vi "Target.vi"() -> ()   [LabVIEW 2018]
uses:
  <vilib>/Platform/TimedLoop/XDataNode/timing_clust.ctl
  <vilib>/Platform/TimedLoop/XDataNode/nitl_modes.ctl
  <vilib>/Platform/TimedLoop/XDataNode/wakeup.ctl
  <vilib>/rvi/eio/common/nirviEmuTemplateMethod_errors.vi
  <vilib>/rvi/Emulation/niFpgaGetClockAttributes.vi
  <vilib>/rvi/Emulation/niFpgaSctlEmulationGetInTimedLoop.vi
  <vilib>/rvi/Emulation/niFpgaEmulationReportErrorSimple.vi
  <vilib>/rvi/Emulation/niFpgaCriticalErrorInLSC.vi
  <vilib>/rvi/Emulation/niFpgaProcessEmulError.vi
  <vilib>/rvi/DataTransferAndStorage/Container/Common/niFpgaContainerGetUniqueNameForEmu.vi
  <vilib>/rvi/interface/RandomDataEmulation/niFpgaRandomDataHandleErrors.vi
  <vilib>/rvi/Memory/Memory_Emulation/niFpgaMemoryFastEmulationDramWriteAndRequestData.vi
  <vilib>/rvi/Memory/Memory_Emulation/niFpgaMemoryEmulationDramWriteAndRequestData.vi
  <vilib>/rvi/Memory/Memory_Emulation/niFpgaMemoryEmulationDramWriteAndRequestDataApplyByteEnables.vi
  <vilib>/eio/EIONode/EIONode.xnode
  <vilib>/Platform/TimedLoop/XDataNode/XDataNode.xnode
  <vilib>/rvi/DataTransferAndStorage/Container/XNode/niFpgaContainer.xnode
  <vilib>/rvi/Memory/Memory_Emulation/niFpgaMemoryEmulationDramRetrieveData.vi
  <vilib>/rvi/interface/RandomDataEmulation/nirviRandomDataFpgaReadWriteTemplate.vi
  <vilib>/Platform/TimedLoop/XDataNode/XDNodeRunTimeDep.lvlib
panel:
  in  "TrigTime":u32=500
  in  "ForcedStopMemory":bool
  out "CountFIFO":u32
  out "AddCounter":u32
  in  "9..0(F)/0..9(T)":bool
  in  "Retrieve":u8=1
  in  "Request":u8
  in  "ResetFIFO":bool
  out "FIFOIsDone":bool
  in  "ResetMemory":bool
  out "MemoryIsDone":bool
  in  "LastAdd":u32=81920
  in  "FirstAdd":u32
  in  "MemoryToFIFO":bool
  in  "DataToMemory":bool
  in  "NumberOfAdd":u32=1310720
  in  "18_STOP":u8=18
  in  "26_STOP":u8=26
  in  "TRIG":bool
  in  "Такт чтения после адреса":u8
  in  "Чтение по С(F)/Ф(T)":bool
  in  "CSN в конце по С(F)/Ф(T)":bool
  in  "ResetSPI":bool
  out "SPI_is_done":bool
  in  "Делитель 24/x":u8=2
  in  "Автомат":bool
  in  "RESET":bool
  out "MISO":bool[](array[boolean])
  in  "MOSI":bool[](array[boolean])=[FALSE, FALSE, FALSE, FALSE, FALSE, FALSE, FALSE, FALSE, FALSE, FALSE, FALSE, FALSE, FALSE, FALSE, FALSE, FALSE, FALSE, FALSE, FALSE, FALSE, FALSE, FALSE, FALSE, FALSE]
  in  "SPI":bool
  in  "8-bit(F)/16-bit(T)":bool
  in  "Stop_FPGA":bool
  # "0"
  # "0"
  # "7"
  # "7"
  # "Начало слова (8 bit)"
  # "Конец адреса (8 bit)"
  # "8"
  # "Начало адреса (8 bit)"
  # "14"
  # "15"
  # "R(F)/W(T) (8 bit)"
  # "Начало слова (16 bit)"
  # "15"
  # "Конец адреса (16 bit)"
  # "16"
  # "Начало адреса (16 bit)"
  # "22"
  # "R(F)/W(T) (16 bit)"
  # "23"
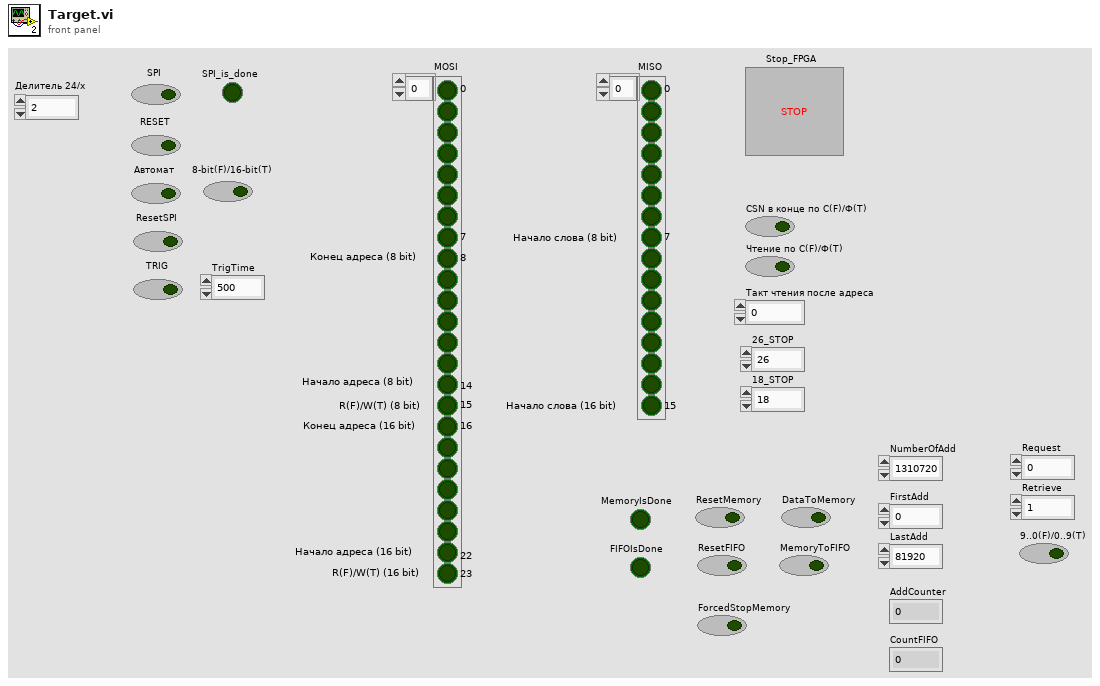
[diagram p1: front panel]
types:
  T1 = typedef "XDNodeRunTimeDep.lvlib/timing_clust.ctl" = cluster{"Expected End [f-1]":u64, "Actual End [f-1]":u64, "Finished Late? [f-1]":bool, "Expected End [i-1]":u64, "Actual End [i-1]":u64, "Finished Late? [i-1]":bool, "Expected Start [i]":u64, "Actual Start [i]":u64, "Expected Start [f]":u64, "Actual Start [f]":u64, "Source Name":string, "Structure Name":string, "Period":i64, "Deadline":i64, "Offset":i64, "Start":i64, "Priority":i32, "Timeout":i32, "Mode":T2, "Wakeup Reason":T3, "Error":errorcluster, "Source Type":string, "Secondary Source Type":string, "Global End Time":u64, "Global Start Time":u64, "Frame Duration":u64, "Iteration Duration":u64, "Assigned CPU":i32, "I/O Scan Engine Mode":u32}
  T2 = typedef "XDNodeRunTimeDep.lvlib/nitl_modes.ctl" = enum32{"No Change", "Process missed periods, maintain original phase", "Discard missed periods, maintain original phase", "Process missed periods, ignore original phase", "Discard missed periods, ignore original phase"}
  T3 = typedef "XDNodeRunTimeDep.lvlib/wakeup.ctl" = enum32{"Normal", "Aborted", "Asynchronous wakeup", "Timing source error", "Timed loop error", "Timeout"}
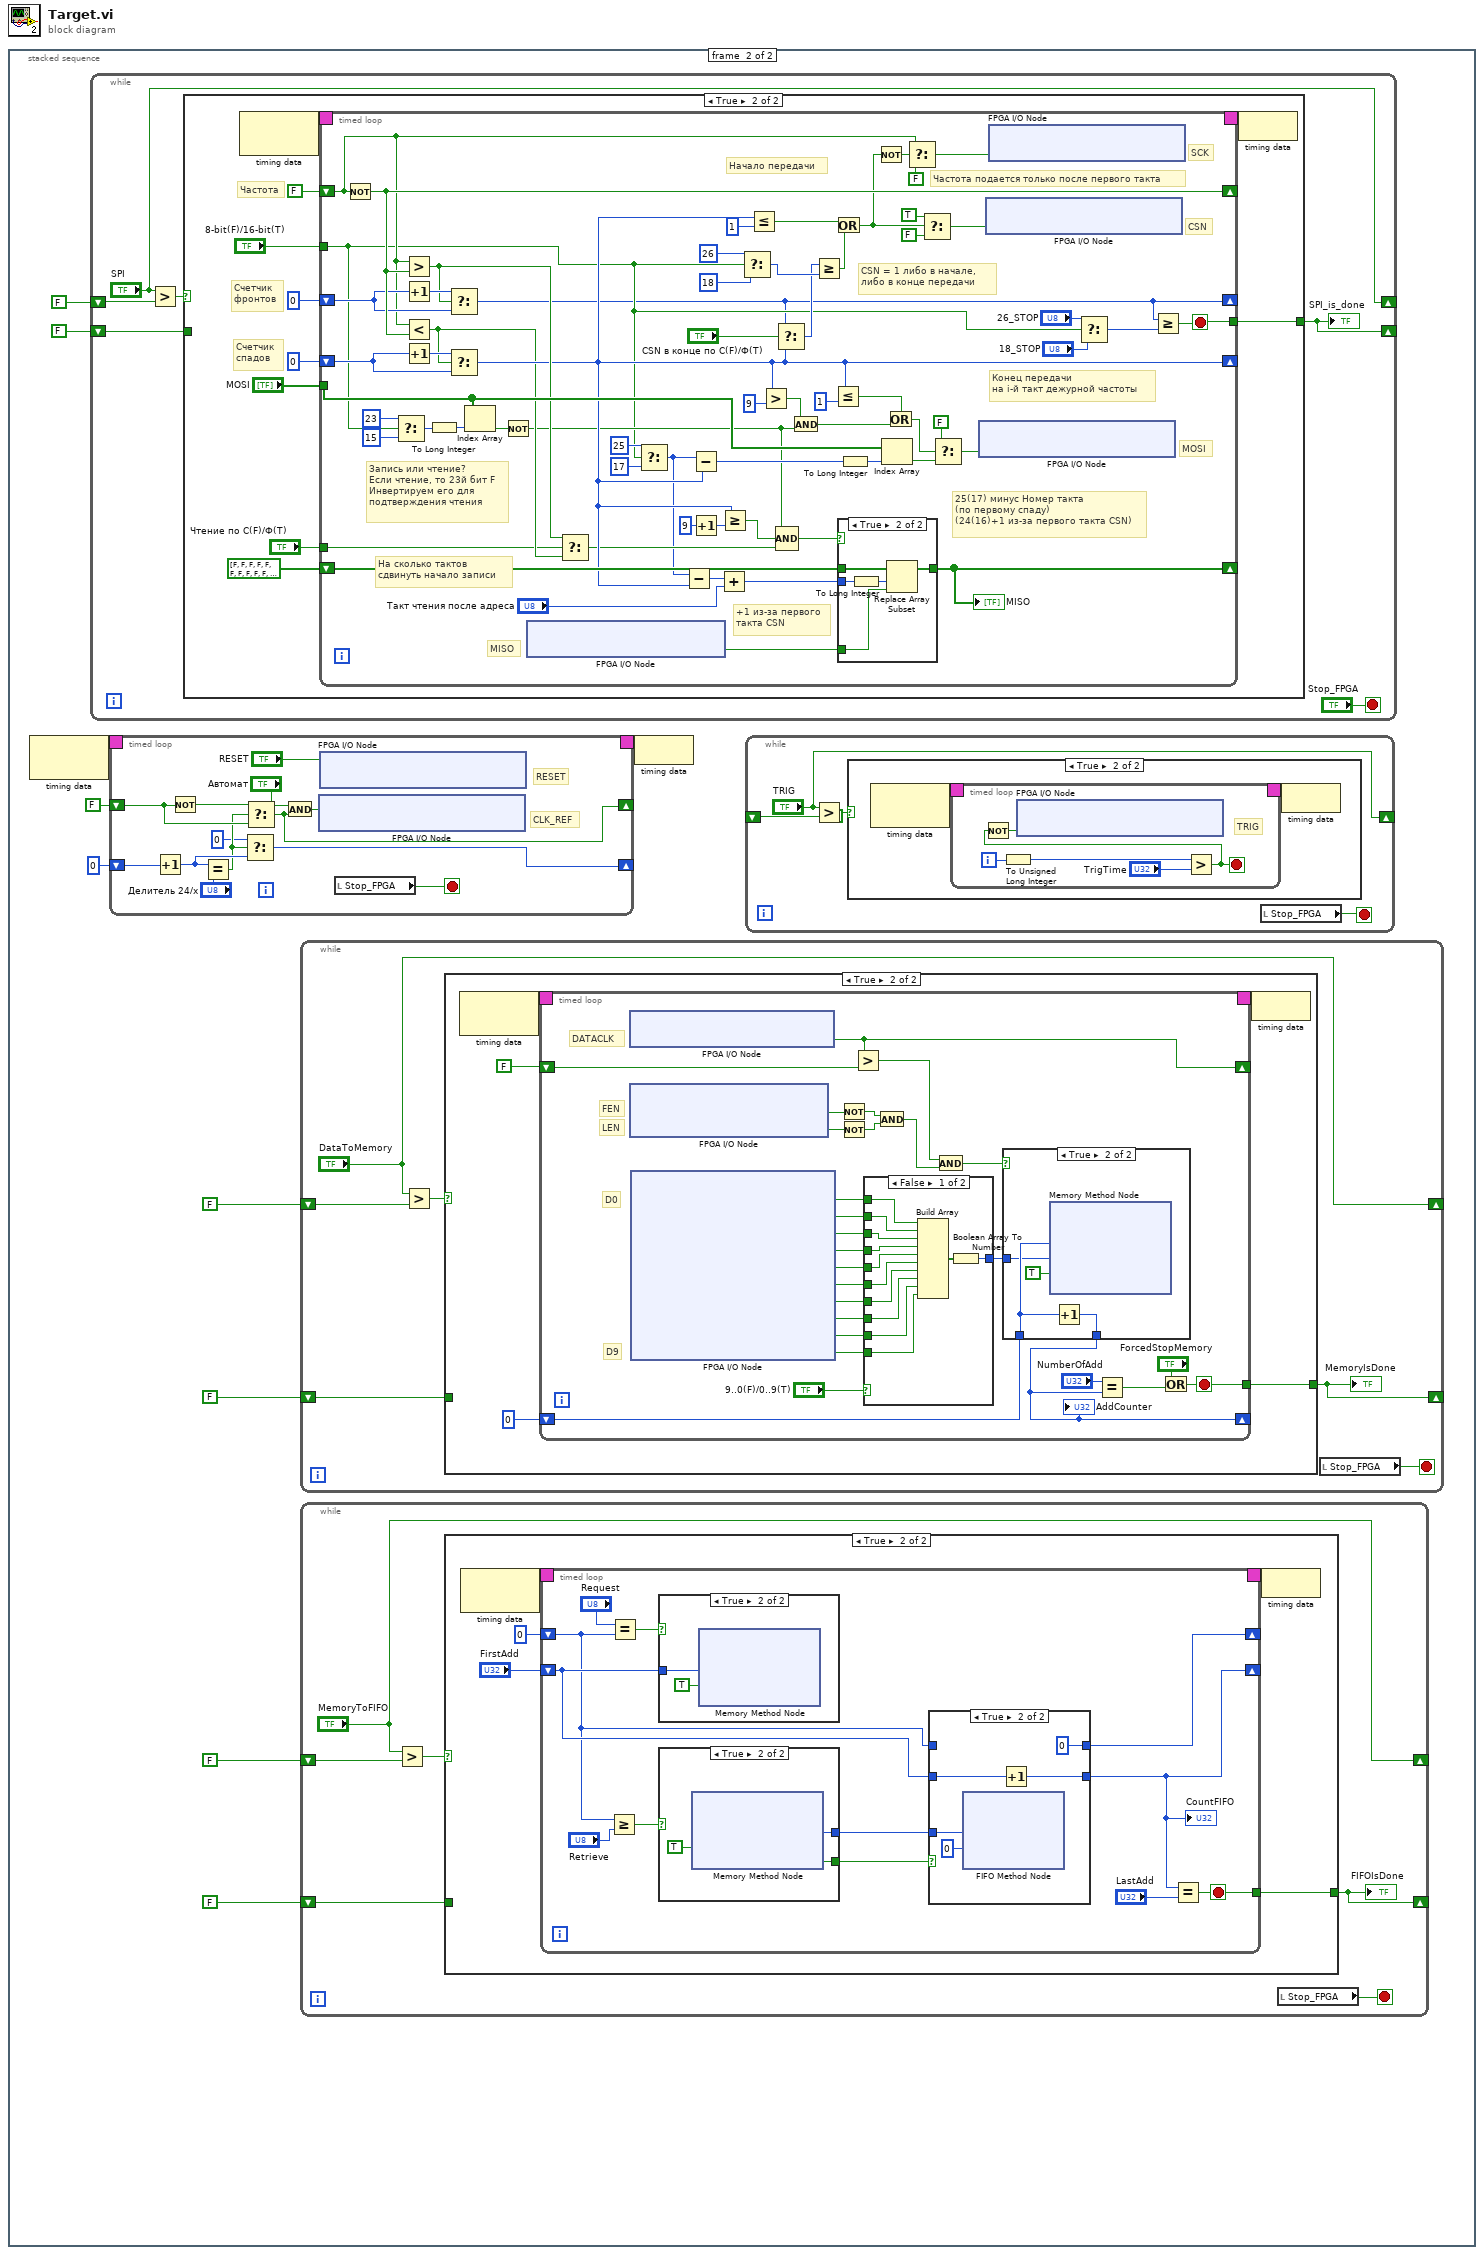
[diagram p0: block diagram]
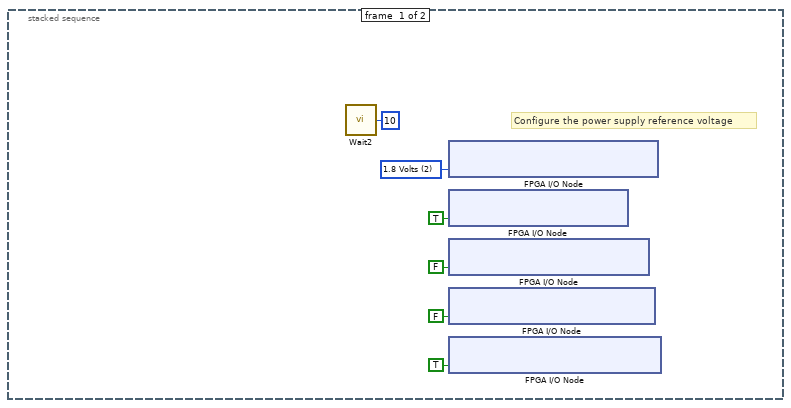
[diagram p2: hidden frame]
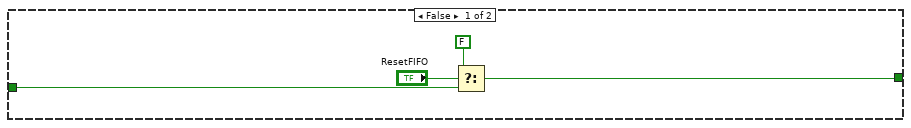
[diagram p4: hidden frame]
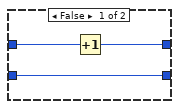
[diagram p5: hidden frame]
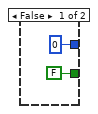
[diagram p6: hidden frame]
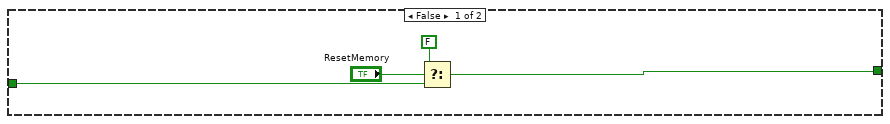
[diagram p8: hidden frame]
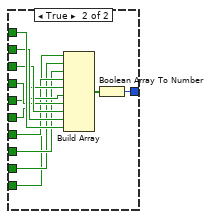
[diagram p9: hidden frame]
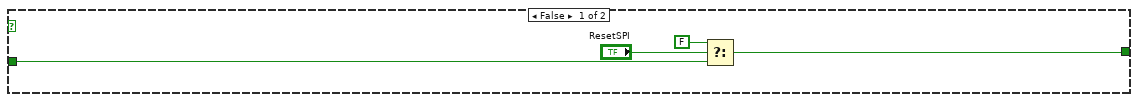
[diagram p11: hidden frame]
diagram:
  n1 = stacked-sequence {
    frame #0 {
      w6 = u8 2 items=["3.3 Volts", "2.5 Volts", "1.8 Volts"] ("Internal Power Supply Voltage")
      # "Configure the power supply reference voltage"
      n2 = call "Wait2"("Count(mSec)"=u8 10) -> ()  [unwired: 1 out]
      n3 = xnode "FPGA I/O Node"("IO Module\\Local_Supply_Select"=w6) -> ()  [unwired: 1 in, 1 out]
      n4 = xnode "FPGA I/O Node"("IO Module\\DDCA_PFI_WE"=TRUE ("IO Module\\DDCB_PFI_WE")) -> ()  [unwired: 1 in, 1 out]
      n5 = xnode "FPGA I/O Node"("IO Module\\DDCA_DIO0-7_WE"=FALSE ("IO Module\\DDCA_DIO0-7_WE")) -> ()  [unwired: 1 in, 1 out]
      n6 = xnode "FPGA I/O Node"("IO Module\\DDCA_DIO8-15_WE"=FALSE ("IO Module\\DDCA_DIO8-15_WE")) -> ()  [unwired: 1 in, 1 out]
      n7 = xnode "FPGA I/O Node"("IO Module\\DDCA_DIO16-23_WE"=TRUE ("IO Module\\DDCA_DIO16-23_WE")) -> ()  [unwired: 1 in, 1 out]
    }
    frame #1 {
      n8 = node-c288() -> (w16:T1)  [unwired: 1 in]
      n9 = while {
        shift-right: ["SPI"] -> _
        shift-left: FALSE -> [w176]
        shift-right: [w171] -> _
        shift-left: FALSE -> [w172]
        stop <- "Stop_FPGA" stop-if-true
        n10 = Greater?(x="SPI", y=w176) -> (0:w175:bool)
        n11 = case shown="True" w175 {
          tunnel: [w179 w185] -> w171
          tunnel: w172 -> [w177 _]
          frame False {
            n12 = Select(t=FALSE, s="ResetSPI", f=w177) -> (s? t:f=w179:bool)
          }
          frame True {
            # "Счетчик\nфронтов"
            # "Счетчик\nспадов"
            # "Частота"
            n13 = node-c288() -> (w190:T1)  [unwired: 1 in]
            n14 = timed-loop {
              timing: w190 -> [_]
              timing-out: [_] -> w189
              shift-right: [w196] -> _
              shift-left: u8 0 -> [w249]
              shift-right: [w252] -> _
              shift-left: FALSE -> [w244]
              shift-right: [w219] -> _
              shift-left: u8 0 -> [w250]
              tunnel: [w195] -> w185
              tunnel: "8-bit(F)/16-bit(T)" -> [w198]
              shift-right: [w233] -> _
              shift-left: bool[] [FALSE, FALSE, FALSE, FALSE, FALSE, FALSE, FALSE, FALSE, FALSE, FALSE, FALSE, FALSE, FALSE, FALSE, FALSE, FALSE] -> [w234]
              tunnel: "MOSI" -> [w228]
              tunnel: "Чтение по С(F)/Ф(T)" -> [w204]
              stop <- w195 stop-if-true
              # "MISO"
              # "MOSI"
              # "CSN"
              # "SCK"
              # "На сколько тактов \ncдвинуть начало записи"
              # "25(17) минус Номер такта\n(по первому спаду)\n(24(16)+1 из-за первого такта CSN)"
              # "Запись или чтение?\nЕсли чтение, то 23й бит F\nИнвертируем его для\nподтверждения чтения"
              # "+1 из-за первого\nтакта CSN"
              # "Конец передачи\nна i-й такт дежурной частоты"
              # "Начало передачи"
              # "Частота подается только после первого такта"
              # "CSN = 1 либо в начале,\nлибо в конце передачи"
              n15 = Not(x=w244) -> (.not. x?=w252:bool)
              n16 = Select(t=u8 23, s=w198, f=u8 15) -> (s? t:f=w241:u8)
              n17 = Greater?(x=w244, y=w252) -> (0:w222:bool)
              n18 = Increment(x=w249) -> (x+1=w253:u8)
              n19 = Less?(x=w244, y=w252) -> (x < y?=w214:bool)
              n20 = Increment(x=w250) -> (x+1=w251:u8)
              n21 = To Long Integer(number=w241) -> (32bit integer=w240:i32)
              n22 = Select(t=w253, s=w222, f=w249) -> (s? t:f=w196:u8)
              n23 = Select(t=w251, s=w214, f=w250) -> (s? t:f=w219:u8)
              n24 = Index Array(array=w228, index=w240) -> (element=w218:bool)
              n25 = Not(x=w218) -> (.not. x?=w212:bool)
              n26 = xnode "FPGA I/O Node"() -> ("IO Module\\DDCA_DIO0_Read"=w191:bool)  [unwired: 1 in, 1 out]
              n27 = Select(t=w222, s=w204, f=w214) -> (s? t:f=w213:bool)
              n28 = Select(t=u8 25 ("y"), s=w198, f=u8 17) -> (s? t:f=w209:u8)
              n29 = Subtract(x=w209, y=w219) -> (x-y=w203:u8)
              n30 = Subtract(x=w209, y=w219) -> (x-y=w221:u8)
              n31 = Increment(x=u8 9 ("Такт чтения")) -> (x+1=w215:u8)
              n32 = Add(x=w203, y="Такт чтения после адреса") -> (x+y=w220:u8)
              n33 = Greater Or Equal?(x=w219, y=w215) -> (x >= y?=w217:bool)
              n34 = Select(t=u8 26 ("Такт CSN в коцне"), s=w198, f=u8 18 ("Такт CSN в конце")) -> (s? t:f=w208:u8)
              n35 = Less Or Equal?(x=w219, y=u8 1 ("1")) -> (x <= y?=w245:bool)
              n36 = Greater?(x=w219, y=u8 9 ("18")) -> (0:w236:bool)
              n37 = Select(t=w196, s="CSN в конце по С(F)/Ф(T)", f=w219) -> (s? t:f=w207:u8)
              n38 = Compound Arithmetic op=AND(w212, w217, w213) -> (w237:bool)
              n39 = And(x=w236, y=w212) -> (x .and. y?=w232:bool)
              n40 = Greater Or Equal?(x=w207, y=w208) -> (x >= y?=w201:bool)
              n41 = Less Or Equal?(x=w219, y=u8 1 ("18")) -> (x <= y?=w230:bool)
              n42 = Or(x=w245, y=w201) -> (x .or. y?=w205:bool)
              n43 = case shown="True" w237 {
                tunnel: w220 -> [_ w259]
                tunnel: w234 -> [w254 w258]
                tunnel: [w254 w257] -> w233
                tunnel: w191 -> [_ w255]
                frame False {
                }
                frame True {
                  n44 = To Long Integer(number=w259) -> (32bit integer=w256:i32)
                  n45 = Replace Array Subset(array=w258, new element=w255, index=w256) -> (w257:bool[])
                }
              }
              "MISO" <- w233
              n46 = To Long Integer(number=w221) -> (32bit integer=w248:i32)
              n47 = Not(x=w205) -> (.not. x?=w206:bool)
              n48 = Index Array(array=w228, index=w248) -> (element=w239:bool)
              n49 = Or(x=w230, y=w232) -> (x .or. y?=w231:bool)
              n50 = Select(t=w244, s=w206, f=FALSE) -> (s? t:f=w194:bool)
              n51 = Select(t=TRUE, s=w205, f=FALSE) -> (s? t:f=w193:bool)
              n52 = Select(t=FALSE, s=w231, f=w239) -> (s? t:f=w192:bool)
              n53 = xnode "FPGA I/O Node"("IO Module\\DDCA_PFI3_Write"=w192) -> ()  [unwired: 1 in, 1 out]
              n54 = xnode "FPGA I/O Node"("IO Module\\DDCA_PFI2_Write"=w193) -> ()  [unwired: 1 in, 1 out]
              n55 = xnode "FPGA I/O Node"("IO Module\\DDCA_PFI1_Write"=w194) -> ()  [unwired: 1 in, 1 out]
              n56 = Select(t="26_STOP", s=w198, f="18_STOP") -> (s? t:f=w197:u8)
              n57 = Greater Or Equal?(x=w196, y=w197) -> (x >= y?=w195:bool)
            }
            n58 = node-c288(w189) -> ()
          }
        }
        "SPI_is_done" <- w171
      }
      n59 = timed-loop {
        timing: w16 -> [_]
        timing-out: [_] -> w15
        shift-right: [w155] -> _
        shift-left: FALSE -> [w164]
        shift-right: [w156] -> _
        shift-left: u8 0 -> [w161]
        stop <- w154 stop-if-true
        # "CLK_REF"
        # "RESET"
        n60 = Increment(x=w161) -> (x+1=w159:u8)
        n61 = Not(x=w164) -> (.not. x?=w165:bool)
        n62 = Equal?(x=w159, y="Делитель 24/x") -> (x = y?=w158:bool)
        n63 = Select(t=u8 0, s=w158, f=w159) -> (s? t:f=w156:u8)
        n64 = Select(t=w165, s=w158, f=w164) -> (s? t:f=w155:bool)
        n65 = And(x="Автомат", y=w155) -> (x .and. y?=w163:bool)
        n66 = xnode "FPGA I/O Node"("IO Module\\DDCA_DIO16_Write"=w163) -> ()  [unwired: 1 in, 1 out]
        n67 = xnode "FPGA I/O Node"("IO Module\\DDCA_DIO19_Write"="RESET") -> ()  [unwired: 1 in, 1 out]
        n68 = local read "Stop_FPGA"() -> (w154:bool)
      }
      n69 = while {
        shift-right: ["DataToMemory"] -> _
        shift-left: FALSE -> [w83]
        shift-right: [w79] -> _
        shift-left: FALSE -> [w80]
        stop <- w84 stop-if-true
        n70 = Greater?(x="DataToMemory", y=w83) -> (0:w82:bool)
        n71 = case shown="True" w82 {
          tunnel: [w86 w89] -> w79
          tunnel: w80 -> [w85 _]
          frame False {
            n72 = Select(t=FALSE, s="ResetMemory", f=w85) -> (s? t:f=w86:bool)
          }
          frame True {
            n73 = node-c288() -> (w93:T1)  [unwired: 1 in]
            n74 = timed-loop {
              timing: w93 -> [_]
              timing-out: [_] -> w92
              shift-right: [w112] -> _
              shift-left: FALSE -> [w113]
              shift-right: [w99] -> _
              shift-left: u32 0 -> [w111]
              tunnel: [w95] -> w89
              stop <- w95 stop-if-true
              # "D0"
              # "D9"
              # "DATACLK"
              # "LEN"
              # "FEN"
              n75 = xnode "FPGA I/O Node"() -> ("IO Module\\DDCA_DIO15_Read"=w112:bool)  [unwired: 1 in, 1 out]
              n76 = xnode "FPGA I/O Node"() -> ("IO Module\\DDCA_DIO1_Read"=w118:bool, "IO Module\\DDCA_DIO2_Read"=w117:bool)  [unwired: 2 in, 2 out]
              n77 = xnode "FPGA I/O Node"() -> ("IO Module\\DDCA_DIO13_Read"=w110:bool, "IO Module\\DDCA_DIO12_Read"=w109:bool, "IO Module\\DDCA_DIO11_Read"=w108:bool, "IO Module\\DDCA_DIO10_Read"=w107:bool, "IO Module\\DDCA_DIO9_Read"=w106:bool, "IO Module\\DDCA_DIO8_Read"=w105:bool, "IO Module\\DDCA_DIO6_Read"=w104:bool, "IO Module\\DDCA_DIO5_Read"=w103:bool, "IO Module\\DDCA_DIO4_Read"=w102:bool, "IO Module\\DDCA_DIO3_Read"=w101:bool)  [unwired: 10 in, 10 out]
              n78 = Not(x=w118) -> (.not. x?=w119:bool)
              n79 = Not(x=w117) -> (.not. x?=w120:bool)
              n80 = Greater?(x=w112, y=w113) -> (0:w114:bool)
              n81 = case shown="False" "9..0(F)/0..9(T)" {
                tunnel: w110 -> [w132 w144]
                tunnel: w109 -> [w131 w143]
                tunnel: w108 -> [w130 w142]
                tunnel: w107 -> [w129 w141]
                tunnel: w106 -> [w128 w140]
                tunnel: w105 -> [w127 w139]
                tunnel: w104 -> [w126 w138]
                tunnel: w103 -> [w125 w137]
                tunnel: w102 -> [w124 w136]
                tunnel: w101 -> [w123 w135]
                tunnel: [w121 w133] -> w97
                frame False {
                  n82 = Build Array(w132, w131, w130, w129, w128, w127, w126, w125, w124, w123) -> (w122:bool[])
                  n83 = Boolean Array To Number(Boolean array=w122) -> (number=w121:u16)
                }
                frame True {
                  n84 = Build Array(w135, w136, w137, w138, w139, w140, w141, w142, w143, w144) -> (w134:bool[])
                  n85 = Boolean Array To Number(Boolean array=w134) -> (number=w133:u16)
                }
              }
              n86 = And(x=w119, y=w120) -> (x .and. y?=w115:bool)
              n87 = And(x=w114, y=w115) -> (x .and. y?=w116:bool)
              n88 = case shown="True" w116 {
                tunnel: [w145 w148] -> w99
                tunnel: w111 -> [w145 w147]
                tunnel: w97 -> [_ w146]
                frame False {
                }
                frame True {
                  n89 = xnode ("Memory Method Node")("Address"=w147, "Data"=w146, "Input Valid"=TRUE) -> ()  [unwired: 1 in, 2 out]
                  n90 = Increment(x=w147) -> (x+1=w148:u32)
                }
              }
              "AddCounter" <- w99
              n91 = Equal?(x="NumberOfAdd", y=w99) -> (x = y?=w96:bool)
              n92 = Or(x="ForcedStopMemory", y=w96) -> (x .or. y?=w95:bool)
            }
            n93 = node-c288(w92) -> ()
          }
        }
        "MemoryIsDone" <- w79
        n94 = local read "Stop_FPGA"() -> (w84:bool)
      }
      n95 = while {
        shift-right: ["MemoryToFIFO"] -> _
        shift-left: FALSE -> [w37]
        shift-right: [w33] -> _
        shift-left: FALSE -> [w34]
        stop <- w38 stop-if-true
        n96 = Greater?(x="MemoryToFIFO", y=w37) -> (0:w36:bool)
        n97 = case shown="True" w36 {
          tunnel: [w40 w43] -> w33
          tunnel: w34 -> [w39 _]
          frame False {
            n98 = Select(t=FALSE, s="ResetFIFO", f=w39) -> (s? t:f=w40:bool)
          }
          frame True {
            n99 = node-c288() -> (w47:T1)  [unwired: 1 in]
            n100 = timed-loop {
              timing: w47 -> [_]
              timing-out: [_] -> w46
              shift-right: [w51] -> _
              shift-left: u8 0 -> [w49]
              shift-right: [w53] -> _
              shift-left: "FirstAdd" -> [w54]
              tunnel: [w50] -> w43
              stop <- w50 stop-if-true
              n101 = Greater Or Equal?(x=w49, y="Retrieve") -> (x >= y?=w57:bool)
              n102 = Equal?(x="Request", y=w49) -> (x = y?=w59:bool)
              n103 = case shown="True" w59 {
                tunnel: w54 -> [_ w73]
                frame False {
                }
                frame True {
                  n104 = xnode ("Memory Method Node")("Address"=w73, "Input Valid"=TRUE) -> ()  [unwired: 1 in, 2 out]
                }
              }
              n105 = case shown="True" w57 {
                tunnel: [FALSE ("Output Valid") w70] -> w56
                tunnel: [u16 0 ("Data") w71] -> w55
                frame False {
                }
                frame True {
                  n106 = xnode ("Memory Method Node")("Ready for Output"=TRUE) -> ("Data"=w71:u16, "Output Valid"=w70:bool)  [unwired: 1 in, 1 out]
                }
              }
              n107 = case shown="True" w56 {
                tunnel: w55 -> [_ w67]
                tunnel: w54 -> [w62 w65]
                tunnel: [w62 w64] -> w53
                tunnel: [w61 u8 0] -> w51
                tunnel: w49 -> [w60 _]
                frame False {
                  n108 = Increment(x=w60) -> (x+1=w61:u8)
                }
                frame True {
                  n109 = xnode ("FIFO Method Node")("Element"=w67, "Timeout"=0) -> ()  [unwired: 1 in, 2 out]
                  n110 = Increment(x=w65) -> (x+1=w64:u32)
                }
              }
              "CountFIFO" <- w53
              n111 = Equal?(x=w53, y="LastAdd") -> (x = y?=w50:bool)
            }
            n112 = node-c288(w46) -> ()
          }
        }
        "FIFOIsDone" <- w33
        n113 = local read "Stop_FPGA"() -> (w38:bool)
      }
      n114 = node-c288(w15) -> ()
      n115 = while {
        shift-right: ["TRIG"] -> _
        shift-left: FALSE -> [w20]
        stop <- w21 stop-if-true
        n116 = Greater?(x="TRIG", y=w20) -> (0:w19:bool)
        n117 = case shown="True" w19 {
          frame False {
          }
          frame True {
            n118 = node-c288() -> (w23:T1)  [unwired: 1 in]
            n119 = timed-loop {
              timing: w23 -> [_]
              timing-out: [_] -> w22
              i -> [w26]
              stop <- w24 stop-if-true
              # "TRIG"
              n120 = To Unsigned Long Integer(number=w26) -> (unsigned 32bit integer=w28:u32)
              n121 = Greater?(x=w28, y="TrigTime") -> (0:w24:bool)
              n122 = Not(x=w24) -> (.not. x?=w25:bool)
              n123 = xnode "FPGA I/O Node"("IO Module\\DDCA_DIO18_Write"=w25) -> ()  [unwired: 1 in, 1 out]
            }
            n124 = node-c288(w22) -> ()
          }
        }
        n125 = local read "Stop_FPGA"() -> (w21:bool)
      }
    }
  }
